vi "Create Type Definition.vi"(8 "error in (no error)":errorcluster, 11 "library in":refnum<vi>) -> (0 "error out":errorcluster, 2 "TypeDef VI out":refnum<vi>, 3 "library out":refnum<vi>)   [LabVIEW 2019, in "gRPC Template Creation Utility.lvlib"]
uses:
  gRPC Template Creation Utility.lvlib
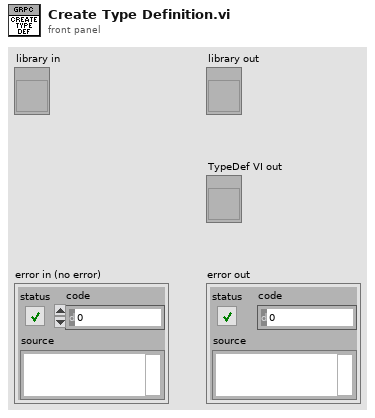
[diagram p1: front panel]
types:
  T1 = enum32{"not a control VI", "control", "typedef", "strict typedef"}
  T2 = enum32{"invalid VI type", "Standard VI", "Control VI", "Global VI", "Polymorphic VI", "Configuration VI", "SubSystem", "Facade VI", "Method VI", "Statechart Diagram VI"}
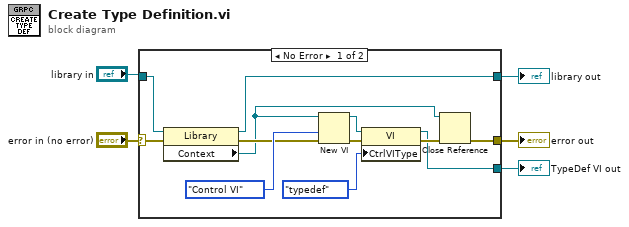
[diagram p0: block diagram]
diagram:
  n1 = case shown="No Error" "error in (no error)" {
    selector: "error in (no error)" -> [w13 w19]
    tunnel: [w9 w19] -> w5
    tunnel: [w10 _] -> w4
    tunnel: "library in" -> [w7 w18]
    tunnel: [w6 w18] -> w1
    frame No Error {
      n2 = property class="Library"(reference=w7, error in=w13) -> (reference out=w6:refnum<vi>, error out=w12:errorcluster, "Context"=w8:refnum<vi>)
      n3 = New VI(8:w12, 9:T2."Control VI" ("vi type (standard vi)"), 11:w8) -> (0:w16:errorcluster, 3:w17:refnum<vi>)  [unwired: 4 in]
      n4 = property class="VI"(reference=w17, error in=w16, "CtrlVIType"=T1."typedef" ("Control VI Type")) -> (reference out=w10:refnum<vi>, error out=w11:errorcluster)
      n5 = Close Reference(reference=w8, error in (no error)=w11) -> (error out=w9:errorcluster)
    }
    frame Error {
    }
  }
  "error out" <- w5
  "TypeDef VI out" <- w4
  "library out" <- w1
